vi "XY Graph Get X Scale Number.vi"(8 "Error In":errorcluster, 11 "XYGraph Ref":T1) -> (0 "Error Out":errorcluster, 2 "# X Scales":i32=1, 3 "XYGraph Ref out":T1)   [LabVIEW 2021, in "XY Graph Add-Ons.lvlib"]
uses:
  XY Graph Add-Ons.lvlib
  XY Graph Refnum.ctl
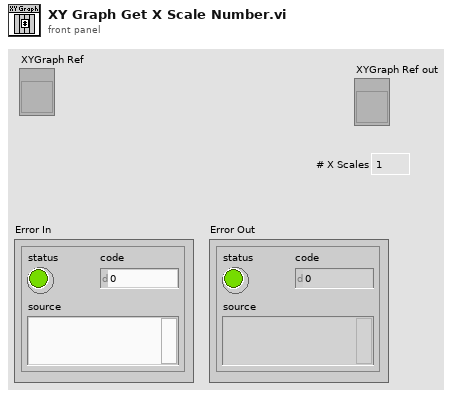
[diagram p1: front panel]
types:
  T1 = typedef "XY Graph Add-Ons.lvlib/XY Graph Refnum.ctl" = refnum<vi>
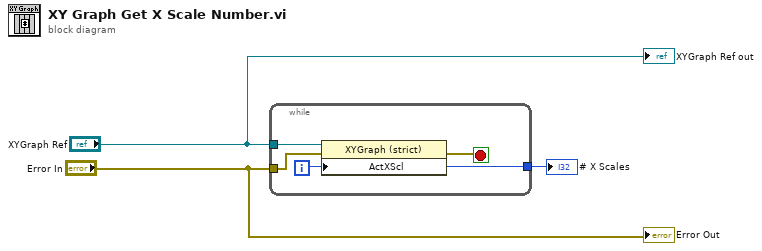
[diagram p0: block diagram]
diagram:
  n1 = while {
    tunnel: "Error In" -> [w6]
    tunnel: "XYGraph Ref" -> [w7]
    tunnel: [w4] -> w2
    i -> [w4]
    stop <- w5 stop-if-true
    n2 = property class="XYGraph (strict)"(reference=w7, error in=w6, "ActXScl"=w4) -> (error out=w5:errorcluster)  [unwired: 1 out]
  }
  "# X Scales" <- w2
  "Error Out" <- "Error In"
  "XYGraph Ref out" <- "XYGraph Ref"
